vi "FdxCmdStrobeTriggerLineCvi.vi"(8 "error in":errorcluster, 10 "TriggerLine":u32(ring) items=["FDX_TX_GENERIC", "FDX_TX_REPLAY", "FDX_TX_INDIVIDUAL"], 11 "InstrumentHandle_board in":u32) -> (0 "error out":errorcluster, 3 "InstrumentHandle_board out":u32)   [LabVIEW 2020, in "AIM664LV.lvlib"]
doc: "This function provides a Trigger output strobe on a selectable Trigger Output Line on system\ncommand."
uses:
  AIM664LV.lvlib
  AFDX_LibraryAdmin/FdxGlobalDllPath.vi
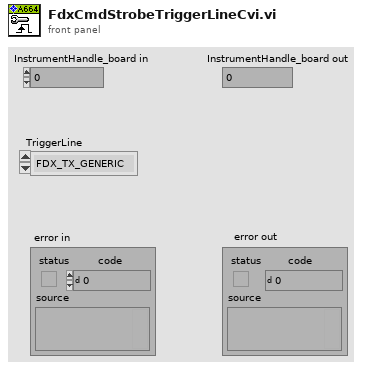
[diagram p1: front panel]
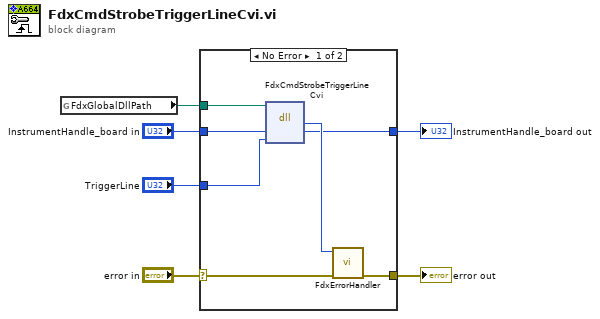
[diagram p0: block diagram]
diagram:
  n1 = global read "FdxGlobalDllPath.vi" "FdxGlobalDllPath"() -> (w4:path)
  n2 = case shown="No Error" "error in" {
    selector: "error in" -> [w12 w15]
    tunnel: [w13 w15] -> w6
    tunnel: w4 -> [w10 _]
    tunnel: "InstrumentHandle_board in" -> [w9 w14]
    tunnel: [w8 w14] -> w2
    tunnel: "TriggerLine" -> [w7 _]
    frame No Error {
      n3 = dll-call lib="aim_fdx.19.dll" fn="FdxCmdStrobeTriggerLineCvi"(path in=w10, "InstrumentHandle"=w9, "TriggerLine"=w7) -> ("status"=w11:i32, "InstrumentHandle"=w8:u32)  [unwired: 3 in, 2 out]
      n4 = call "FdxErrorHandler.vi"("error in"=w12, "AIM Error"=w11) -> ("error out"=w13:errorcluster)  [unwired: 9 in]
    }
    frame Error {
    }
  }
  "error out" <- w6
  "InstrumentHandle_board out" <- w2
